vi "create DAQ strings.vi"(8 "error in (no error)":errorcluster, 11 "MCC USB-DAQ Setup":T1={"Device Name in InstaCal"="Dev0", "Omega Pressure Sensor"={"DAQ Channel"=2.0, "Input Voltage Range"=1, "Enabled"=TRUE, "Description"="Uphole Pressure"}, "McMillian 102 Flowmeter"={"DAQ Channel"=11.0, "Input Voltage Range"=1, "Enabled"=TRUE, "Description"="Flow"}, "DHT Pressure Sensor"={"DAQ Channel"=3.0, "Input Voltage Range"=1, "Enabled"=TRUE, "Description"="Downhole Pressure"}, "Top String Pot"={"DAQ Channel"=0.0, "Input Voltage Range"=0, "Enabled"=TRUE, "Description"="Top String Pot"}, "String Pot Signal"={"DAQ Channel"=1.0, "Input Voltage Range"=0, "Enabled"=TRUE, "Description"="String Pot"}, "Aux Sensor 1"={"DAQ Channel"=5.0, "Input Voltage Range"=1, "Enabled"=FALSE, "Description"="Aux 1"}, "Aux Sensor 2"={"DAQ Channel"=6.0, "Input Voltage Range"=1, "Enabled"=FALSE, "Description"="Aux 2"}, "Aux Sensor 3"={"DAQ Channel"=7.0, "Input Voltage Range"=1, "Enabled"=TRUE, "Description"="Aux 3"}, "Voltage Monitor"={"DAQ Channel"=8.0, "Input Voltage Range"=0, "Enabled"=TRUE, "Description"="9V Monitor"}} {"Voltage Monitor"."Input Voltage Range" items=["+/-10 V Range", "+/-5 V Range", "+/-2.5V Range", "+/-1.25 V Range", "+/-0.625 V Range", "+/-0.3125 V Range", "+/-0.1562V Range", "+/-0.078125 V Range"]; "Aux Sensor 3"."Input Voltage Range" items=["+/-10 V Range", "+/-5 V Range", "+/-2.5V Range", "+/-1.25 V Range", "+/-0.625 V Range", "+/-0.3125 V Range", "+/-0.1562V Range", "+/-0.078125 V Range"]; "Aux Sensor 2"."Input Voltage Range" items=["+/-10 V Range", "+/-5 V Range", "+/-2.5V Range", "+/-1.25 V Range", "+/-0.625 V Range", "+/-0.3125 V Range", "+/-0.1562V Range", "+/-0.078125 V Range"]; "Aux Sensor 1"."Input Voltage Range" items=["+/-10 V Range", "+/-5 V Range", "+/-2.5V Range", "+/-1.25 V Range", "+/-0.625 V Range", "+/-0.3125 V Range", "+/-0.1562V Range", "+/-0.078125 V Range"]; "String Pot Signal"."Input Voltage Range" items=["+/-10 V Range", "+/-5 V Range", "+/-2.5V Range", "+/-1.25 V Range", "+/-0.625 V Range", "+/-0.3125 V Range", "+/-0.1562V Range", "+/-0.078125 V Range"]; "Top String Pot"."Input Voltage Range" items=["+/-10 V Range", "+/-5 V Range", "+/-2.5V Range", "+/-1.25 V Range", "+/-0.625 V Range", "+/-0.3125 V Range", "+/-0.1562V Range", "+/-0.078125 V Range"]; "DHT Pressure Sensor"."Input Voltage Range" items=["+/-10 V Range", "+/-5 V Range", "+/-2.5V Range", "+/-1.25 V Range", "+/-0.625 V Range", "+/-0.3125 V Range", "+/-0.1562V Range", "+/-0.078125 V Range"]; "McMillian 102 Flowmeter"."Input Voltage Range" items=["+/-10 V Range", "+/-5 V Range", "+/-2.5V Range", "+/-1.25 V Range", "+/-0.625 V Range", "+/-0.3125 V Range", "+/-0.1562V Range", "+/-0.078125 V Range"]; "Omega Pressure Sensor"."Input Voltage Range" items=["+/-10 V Range", "+/-5 V Range", "+/-2.5V Range", "+/-1.25 V Range", "+/-0.625 V Range", "+/-0.3125 V Range", "+/-0.1562V Range", "+/-0.078125 V Range"]}) -> (0 "error IO":errorcluster, 1 "Descriptions":string[](array[string]), 2 "delimited string":string, 3 "Array":string[](array[string]), 4 "Voltage Range":dbl[](array[numeric]))   [LabVIEW 2016]
uses:
  controls/Aux Sensor.ctl
  controls/MCC DAQ Setup.ctl
  <vilib>/Utility/VariantDataType/VariantType.lvlib
panel:
  in  "Sensor":T2={"DAQ Channel"=7.0, "Input Voltage Range"=0, "Enabled"=TRUE, "Description"=""} {"Input Voltage Range" items=["+/-10 V Range", "+/-5 V Range", "+/-2.5V Range", "+/-1.25 V Range", "+/-0.625 V Range", "+/-0.3125 V Range", "+/-0.1562V Range", "+/-0.078125 V Range"]}
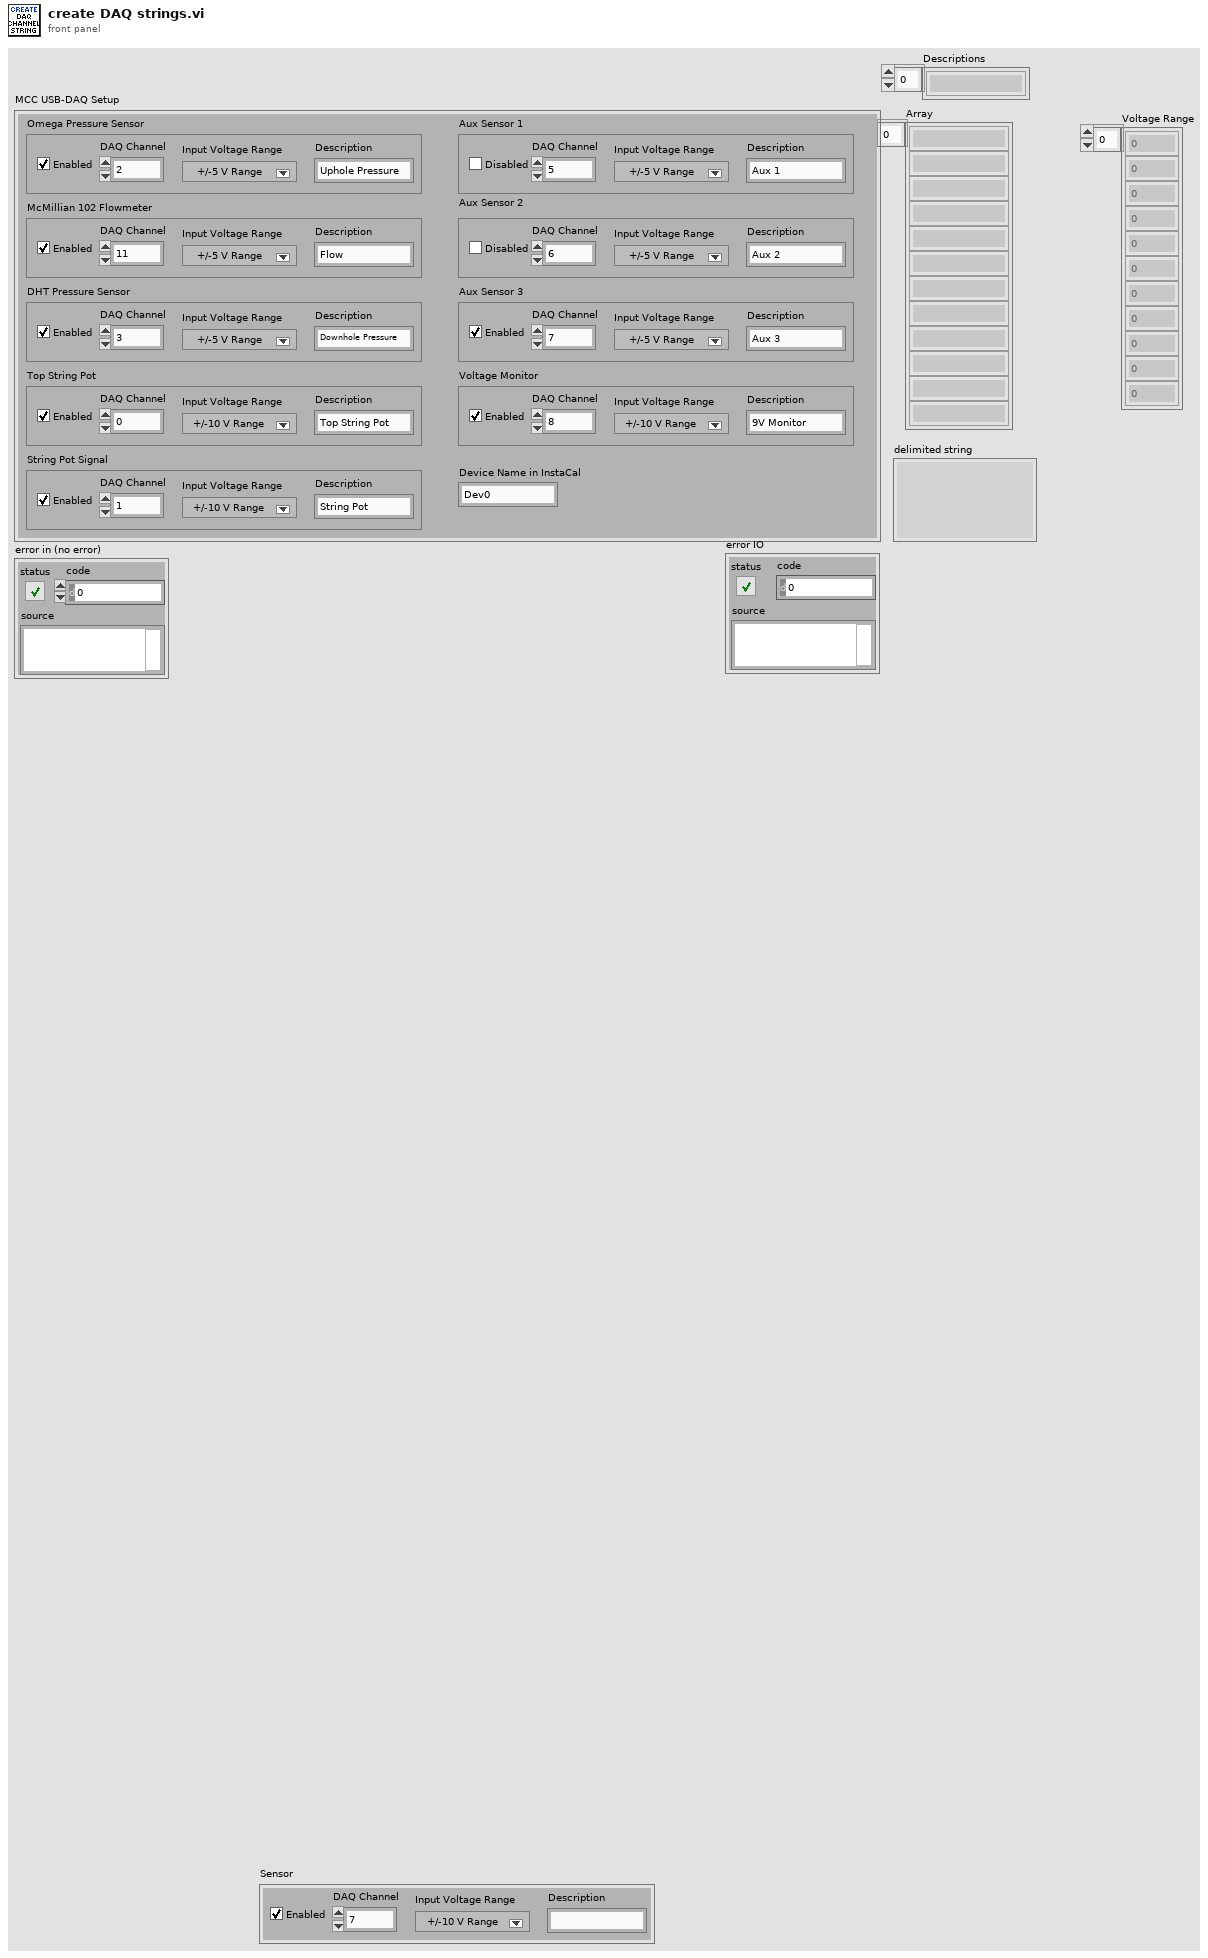
[diagram p1: front panel]
types:
  T1 = typedef "MCC DAQ Setup.ctl" = cluster{"Device Name in InstaCal":string, "Omega Pressure Sensor":T2, "McMillian 102 Flowmeter":T2, "DHT Pressure Sensor":T2, "Top String Pot":T2, "String Pot Signal":T2, "Aux Sensor 1":T2, "Aux Sensor 2":T2, "Aux Sensor 3":T2, "Voltage Monitor":T2}
  T2 = typedef "Aux Sensor.ctl" = cluster{"DAQ Channel":dbl, "Input Voltage Range":u16, "Enabled":bool, "Description":string}
  T3 = typedef "VariantType.lvlib/TypedefInfo.ctl" = cluster{"Name":string, "Timestamp":u32}
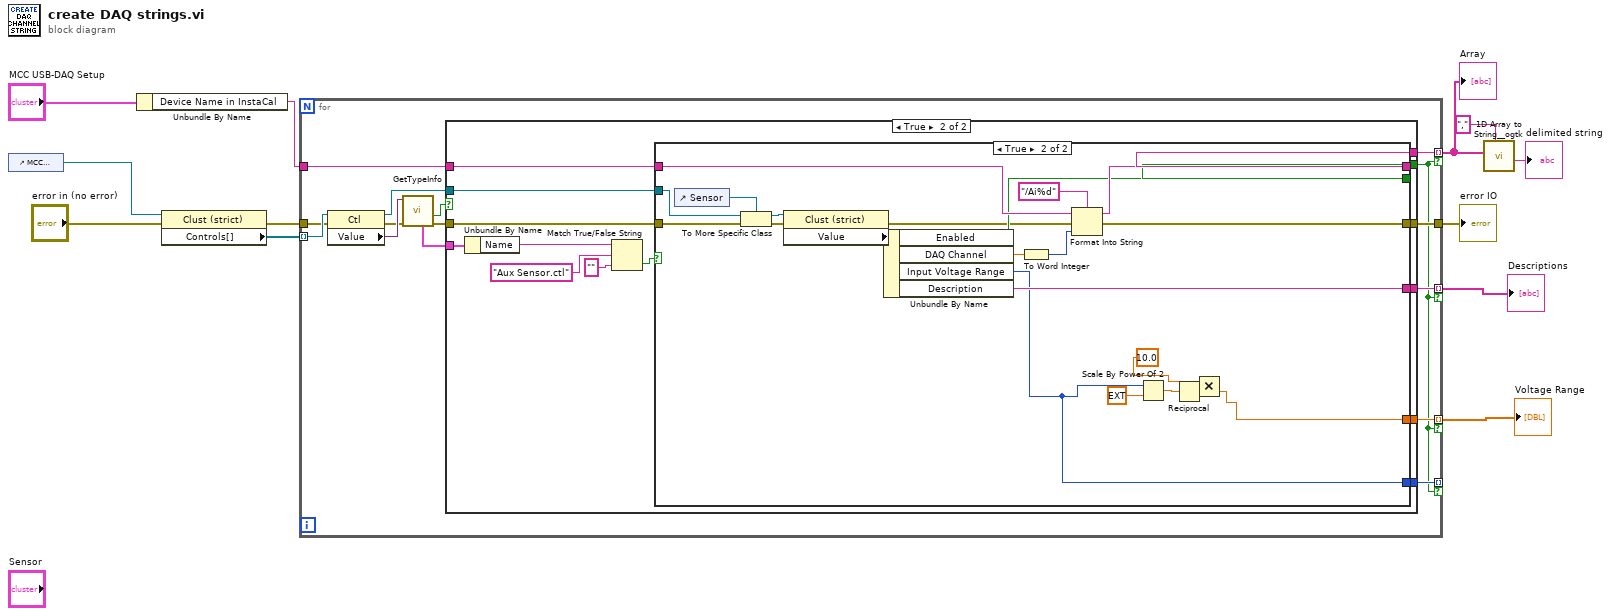
[diagram p0: block diagram]
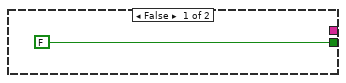
[diagram p2: hidden frame]
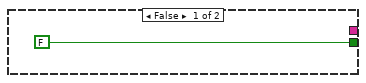
[diagram p3: hidden frame]
diagram:
  n1 = control-ref of="MCC USB-DAQ Setup"() -> (w9:refnum<vi>)
  n2 = Unbundle By Name("MCC USB-DAQ Setup") -> ("Device Name in InstaCal"=w11:string)
  n3 = property class="Clust (strict)"(reference=w9, error in="error in (no error)") -> (error out=w4:errorcluster, "Controls[]"=w12:refnum<vi>[])  [unwired: 1 out]
  n4 = for {
    tunnel: w12 -> [w27] mode=indexing
    tunnel: w11 -> [w22]
    tunnel: [w21] -> w8 mode=indexing if=w13
    tunnel: [w20] -> w5
    tunnel: w4 -> [w17]
    tunnel: [w16] -> w2 mode=indexing if=w13
    tunnel: [w15] -> w1 mode=indexing if=w13
    tunnel: [w14] -> _ mode=indexing if=w13
    n5 = property class="Ctl"(reference=w27, error in=w17) -> (reference out=w23:refnum<vi>, error out=w18:errorcluster, "Value"=w26:variant)
    n6 = call <vilib>:"GetTypeInfo.vi"("error in (no error)"=w18, "Variant"=w26) -> ("error out"=w19:errorcluster, "HasTypedef"=w25:bool, "TypedefInfo"=w24:T3)  [unwired: 5 in, 2 out]
    n7 = case shown="True" w25 {
      tunnel: w24 -> [_ w42]
      tunnel: w23 -> [_ w38]
      tunnel: w22 -> [_ w37]
      tunnel: [_ w36] -> w21
      tunnel: [FALSE ("Enabled") w35] -> w13
      tunnel: [_ w33] -> w20
      tunnel: w19 -> [_ w32]
      tunnel: [_ w31] -> w16
      tunnel: [_ w30] -> w15
      tunnel: [_ w29] -> w14
      frame False {
      }
      frame True {
        n8 = Unbundle By Name(w42) -> ("Name"=w41:string)
        n9 = Match True/False String(2:"" ("false string"), 3:"Aux Sensor.ctl" ("true string"), 4:w41) -> (0:w39:bool)  [unwired: 1 out]
        n10 = case shown="True" w39 {
          tunnel: w38 -> [_ w64]
          tunnel: w37 -> [_ w60]
          tunnel: [_ w57] -> w36
          tunnel: [FALSE ("Enabled") w56] -> w35
          tunnel: [_ w54] -> w33
          tunnel: w32 -> [_ w51]
          tunnel: [_ w50] -> w31
          tunnel: [_ w45] -> w30
          tunnel: [_ w47] -> w29
          frame False {
          }
          frame True {
            n11 = control-ref of="Sensor"() -> (w62:refnum<vi>)
            n12 = To More Specific Class(target class=w62, reference=w64, error in=w51) -> (specific class reference=w63:refnum<vi>, error out=w52:errorcluster)
            n13 = property class="Clust (strict)"(reference=w63, error in=w52) -> (error out=w53:errorcluster, "Value"=w61:T2)  [unwired: 1 out]
            n14 = Unbundle By Name(w61) -> ("Enabled"=w56:bool, "DAQ Channel"=w58:dbl, "Input Voltage Range"=w47:u16, "Description"=w50:string)
            n15 = To Word Integer(number=w58) -> (16bit integer=w55:i16)
            n16 = Format Into String(format string="/Ai%d", initial string=w60, error in=w53, w55) -> (resulting string=w57:string, error out=w54:errorcluster)
            n17 = Scale By Power Of 2(n=w47, x=ext 1.0) -> (x*2^n=w49:ext)
            n18 = Reciprocal(x=w49) -> (1/x=w48:ext)
            n19 = Multiply(x=10.0, y=w48) -> (x*y=w45:ext)
          }
        }
      }
    }
  }
  "Array" <- w8
  "error IO" <- w5
  "Descriptions" <- w2
  "Voltage Range" <- w1
  n20 = call <userlib>:"1D Array to String__ogtk.vi"("delimiter (Tab)"=",", "Array of Strings"=w8) -> ("delimited string"=→"delimited string":string)  [unwired: 9 in]
